vi "EEG.vi"() -> ()   [LabVIEW 2021]
uses:
  <vilib>/Instr/_visa.llb/VISA Configure Serial Port (Instr).vi
panel:
  out "FFT X1 10":cluster{dbl, dbl, dbl[]}(graph)
  out "FFT X7":cluster{dbl, dbl, dbl[]}(graph)
  out "FFT X8":cluster{dbl, dbl, dbl[]}(graph)
  out "FFT X6":cluster{dbl, dbl, dbl[]}(graph)
  out "FFT X5":cluster{dbl, dbl, dbl[]}(graph)
  out "FFT X3":cluster{dbl, dbl, dbl[]}(graph)
  out "Frecuencia Corte Alto":dbl
  in  "Frecuencia Corte Alto":dbl(knob) scale=4.0..45.0
  out "Canal 9":dynamicdata(graph)
  out "Canal 7":dynamicdata(graph)
  out "Canal 8":dynamicdata(graph)
  out "Canal 6":dynamicdata(graph)
  out "Canal 5":dynamicdata(graph) caption="Canal 1"
  out "E9S":dbl[](array[numeric])
  out "E8S":dbl[](array[numeric])
  out "E7S":dbl[](array[numeric])
  out "E6S":dbl[](array[numeric])
  out "E5S":dbl[](array[numeric])
  out "error IO":errorcluster
  out "E4S":dbl[](array[numeric])
  out "E3S":dbl[](array[numeric])
  out "E2S":dbl[](array[numeric])
  out "E1S":dbl[](array[numeric])
  out "DIRECCION 9":string
  out "VALIDADO 2":bool caption="VALIDADO"
  out "FFT X1 4":cluster{dbl, dbl, dbl[]}(graph)
  out "Canal 3":dynamicdata(graph)
  out "Canal 4":dynamicdata(graph)
  out "FFT X4":cluster{dbl, dbl, dbl[]}(graph)
  out "FFT X2":cluster{dbl, dbl, dbl[]}(graph)
  out "Canal 2":dynamicdata(graph)
  out "FFT X1":cluster{dbl, dbl, dbl[]}(graph)
  out "Canal 1":dynamicdata(graph)
  in  "stop":bool
  in  "ADQUIRIR":bool
  out "VALIDADO":bool
  out "DIRECCION 8":string
  out "DIRECCION 7":string
  out "DIRECCION 6":string
  out "DIRECCION 5":string
  out "DIRECCION 4":string
  out "DIRECCION 3":string
  out "DIRECCION 2":string
  out "DIRECCION 1":string
  in  "DETECTAR":bool
  in  "PUERTO COM":refnum<visa-resource-name>
  # "INSTITUTO POLITÉCNICO NACIONAL\nUNIDAD PROFESIONAL INTERDISCIPLINARIA DE INGENIERIA CAMPUS HIDALGO\n\nINTERFAZ EEG"
  # "Direcciones detectadas"
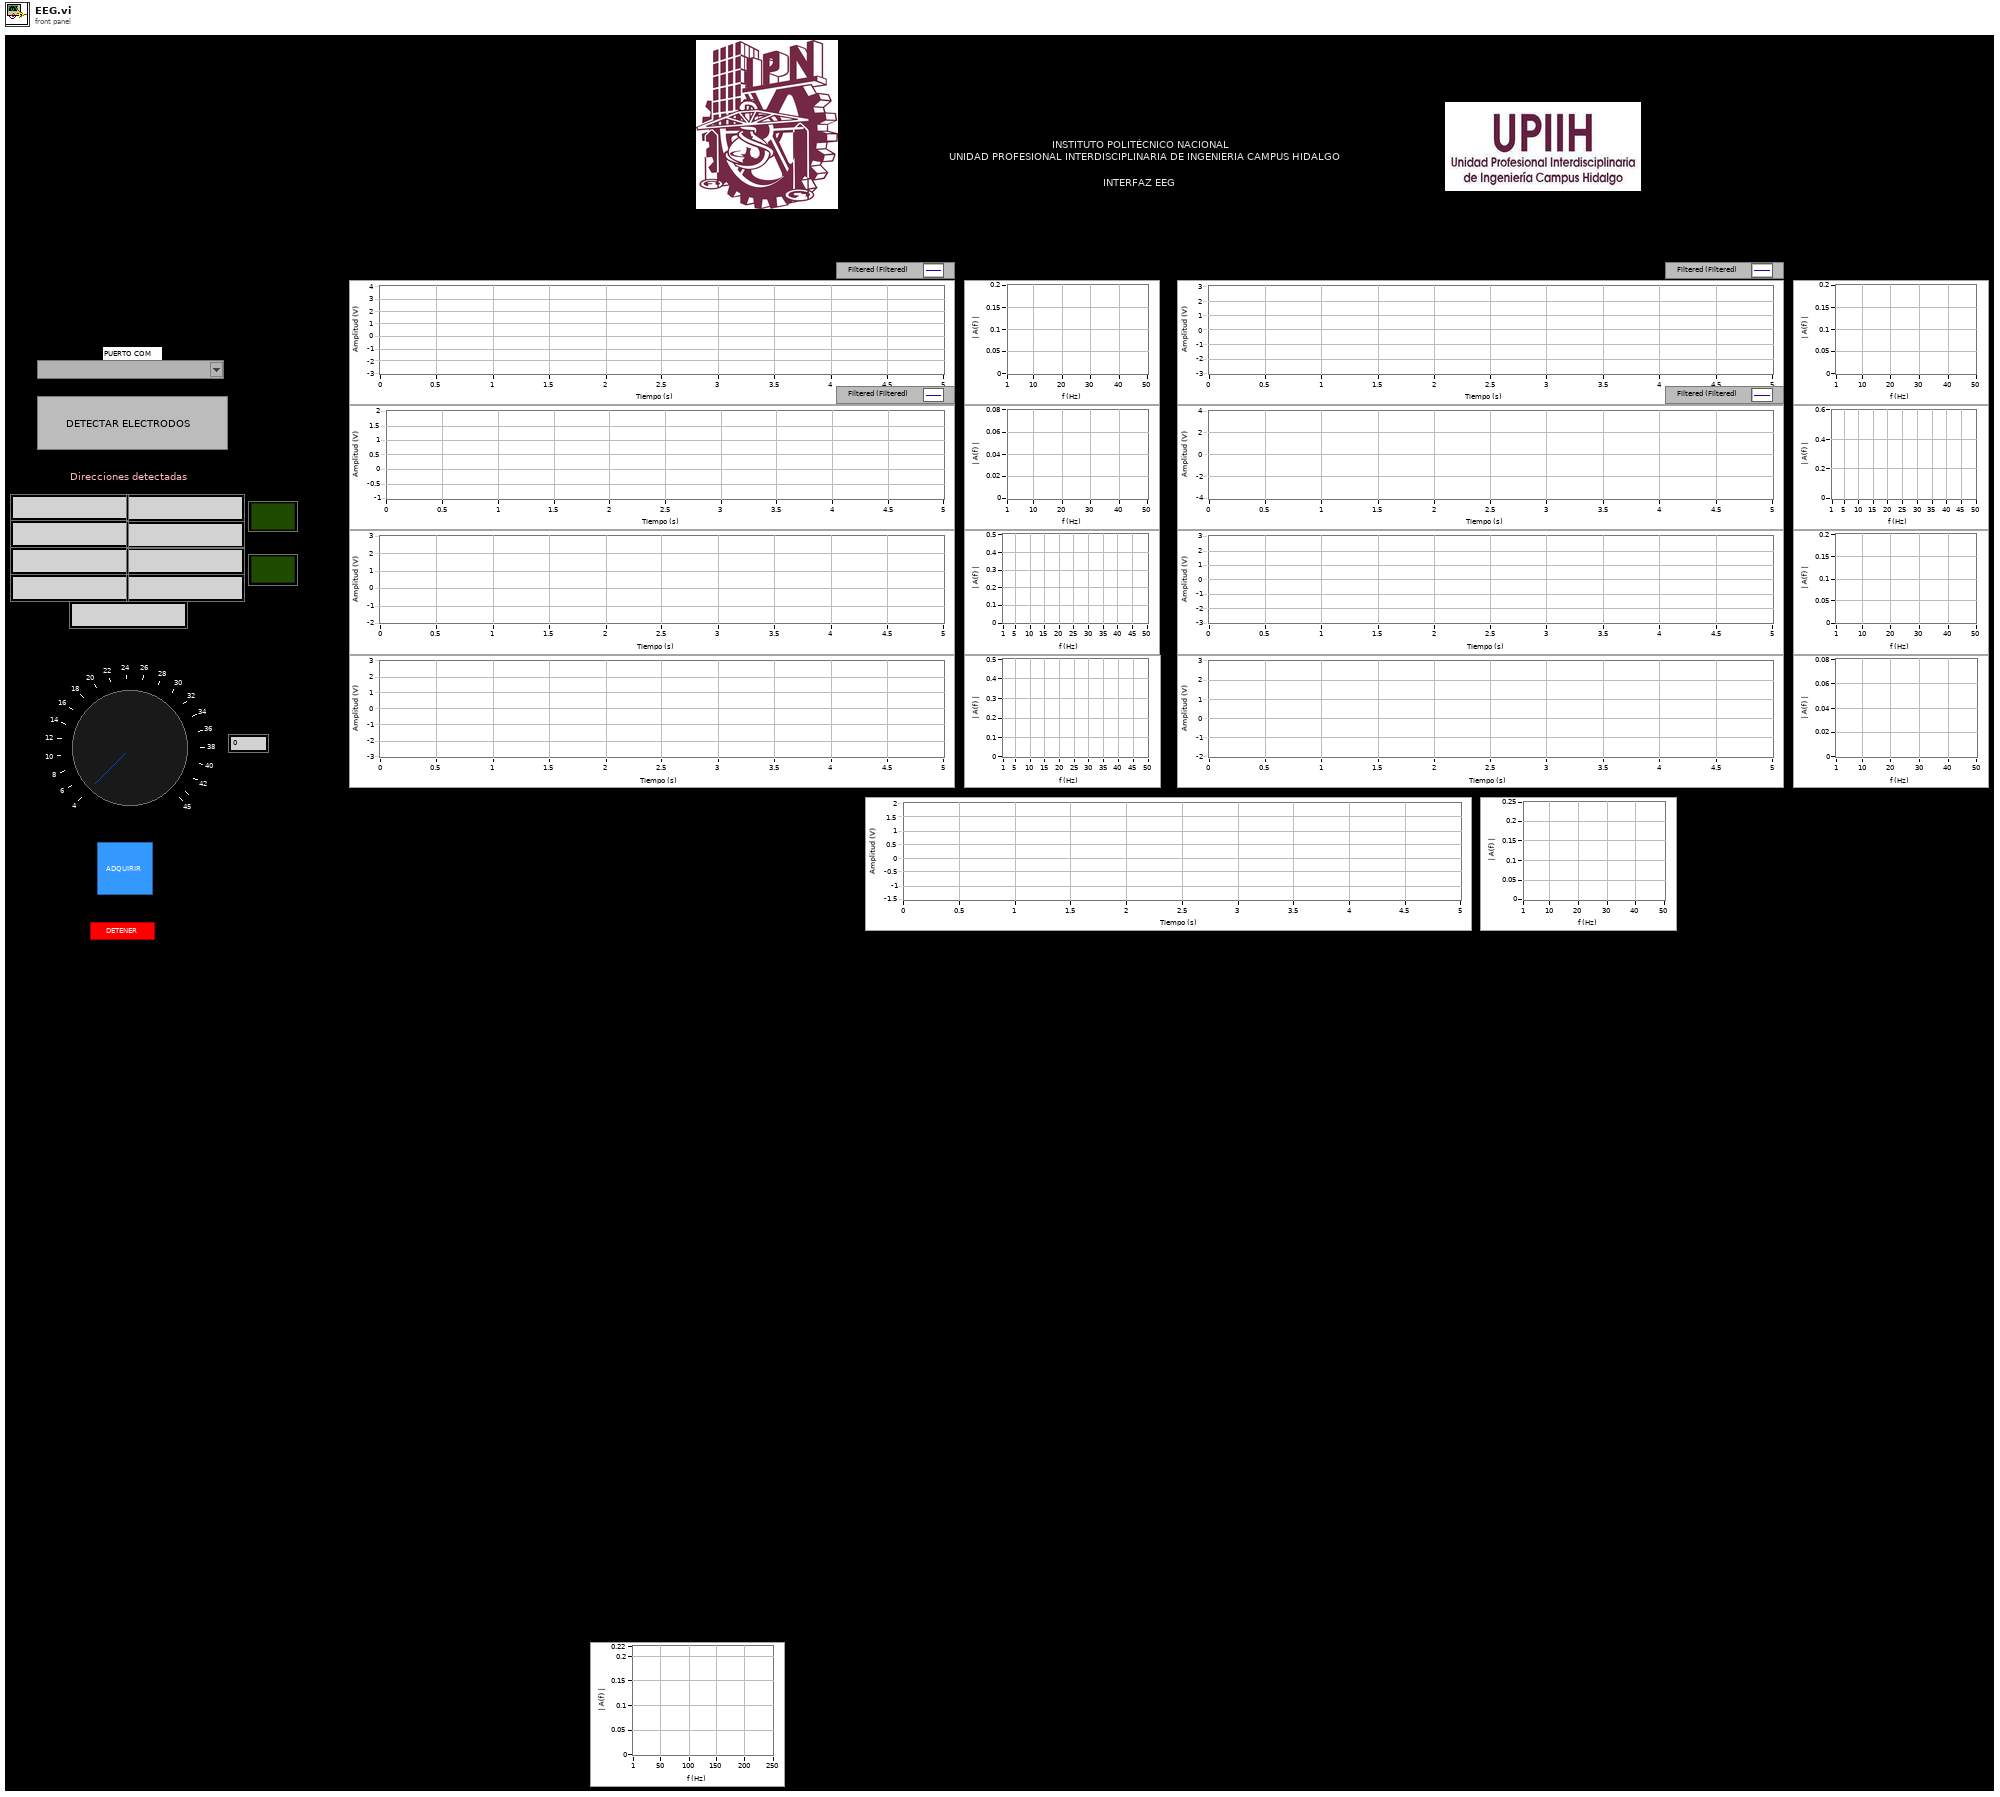
[diagram p1: front panel]
types:
  T1 = cluster{dbl, dbl, dbl, dbl, dbl, dbl, dbl, dbl, dbl}
  T2 = cluster{dbl, dbl, dbl, dbl, dbl, dbl, dbl, dbl, dbl}[]
  T3 = cluster{"Numeric out":dbl, "Numeric 2 out":dbl, "Numeric 3 out":dbl, "Numeric 4 out":dbl, "Numeric 5 out":dbl, "Numeric 6 out":dbl, "Numeric 7 out":dbl, "Numeric 8 out":dbl, "Numeric 9 out":dbl}
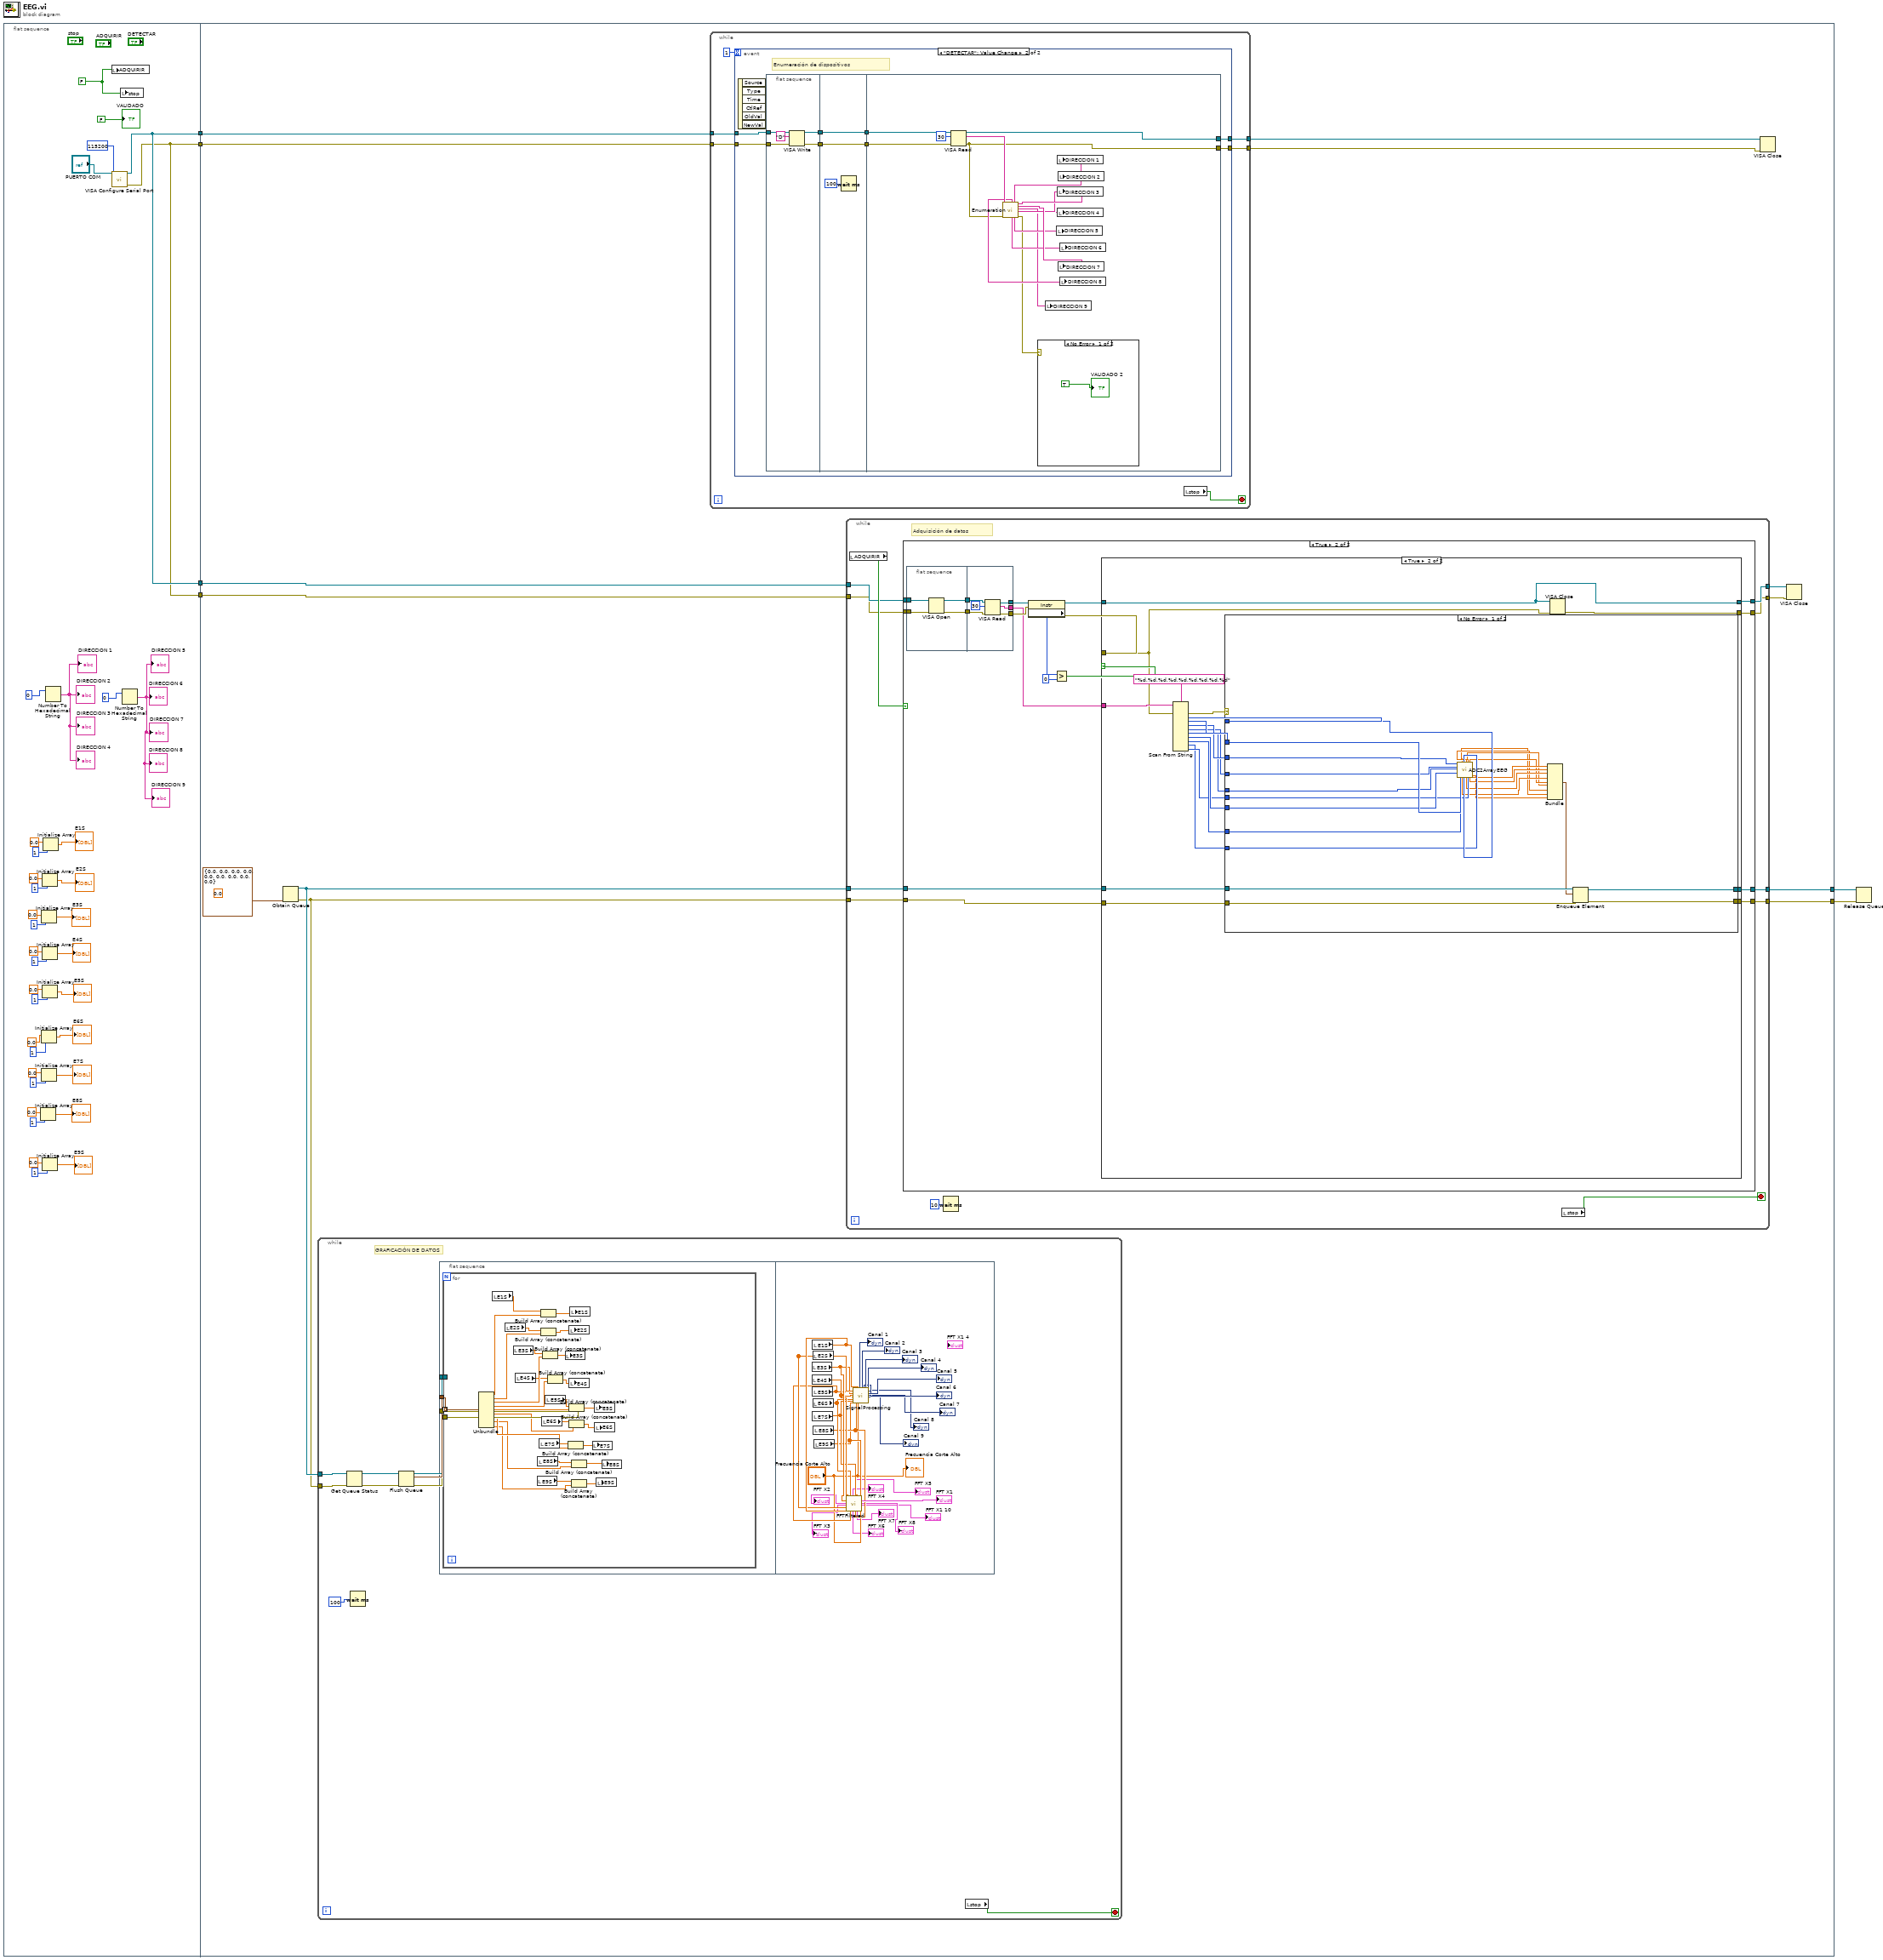
[diagram p0: block diagram]
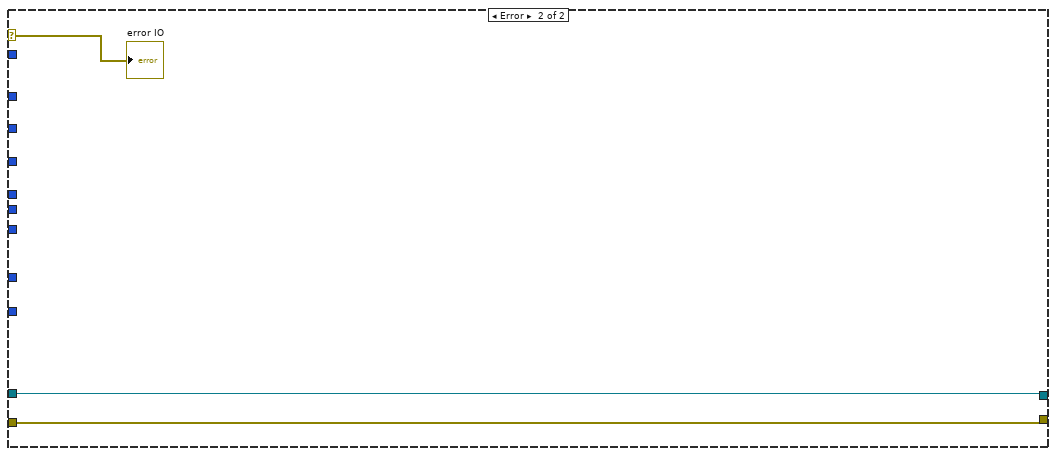
[diagram p4: hidden frame]
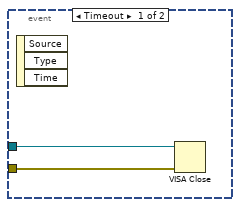
[diagram p5: hidden frame]
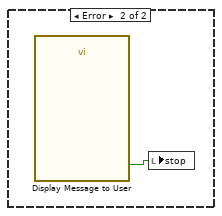
[diagram p6: hidden frame]
diagram:
  n1 = flat-sequence {
    tunnel: [w36] -> w6
    tunnel: [w35] -> w5
    tunnel: [w36] -> w4
    tunnel: [w35] -> w3
    tunnel: w6 -> [w56]
    tunnel: w5 -> [w55]
    tunnel: w4 -> [w52]
    tunnel: w3 -> [w51]
    tunnel: [w48] -> w2
    tunnel: [w47] -> w1
    frame #0 {
      w42 = FALSE
      n2 = Initialize Array(0.0 ("element"), 1 ("dimension size")) -> (→"E8S":dbl[])
      n3 = Initialize Array(0.0 ("element"), 1 ("dimension size")) -> (→"E6S":dbl[])
      n4 = Initialize Array(0.0 ("element"), 1 ("dimension size")) -> (→"E7S":dbl[])
      n5 = Initialize Array(0.0 ("element"), 1 ("dimension size")) -> (→"E3S":dbl[])
      n6 = Initialize Array(0.0 ("element"), 1 ("dimension size")) -> (→"E4S":dbl[])
      n7 = Initialize Array(0.0 ("element"), 1 ("dimension size")) -> (→"E2S":dbl[])
      n8 = Initialize Array(0.0 ("element"), 1 ("dimension size")) -> (→"E5S":dbl[])
      n9 = Initialize Array(0.0 ("element"), 1 ("dimension size")) -> (→"E9S":dbl[])
      n10 = Initialize Array(0.0 ("element"), 1 ("dimension size")) -> (→"E1S":dbl[])
      n11 = Number To Hexadecimal String(2:0) -> (0:→"DIRECCION 3" →"DIRECCION 1" →"DIRECCION 2" →"DIRECCION 4":string)  [unwired: 1 in]
      n12 = local write "ADQUIRIR"(w42) -> ()
      n13 = call-poly "VISA Configure Serial Port"("VISA resource name"="PUERTO COM", "baud rate (9600)"=u32 115200) -> ("VISA resource name out"=w36:refnum<visa-resource-name>, "error out"=w35:errorcluster)  [unwired: 12 in]
      n14 = local write "stop"(w42) -> ()
      n15 = Number To Hexadecimal String(2:0) -> (0:→"DIRECCION 5" →"DIRECCION 6" →"DIRECCION 7" →"DIRECCION 8" →"DIRECCION 9":string)  [unwired: 1 in]
      "VALIDADO" <- FALSE
    }
    frame #1 {
      (unwired) 0.0
      n16 = Obtain Queue(element data type=T1 {0.0, 0.0, 0.0, 0.0, 0.0, 0.0, 0.0, 0.0, 0.0}) -> (queue out=w45:refnum<queue>, error out=w44:errorcluster)  [unwired: 4 in, 1 out]
      n17 = while {
        tunnel: w45 -> [w64]
        tunnel: w44 -> [w63]
        stop <- w65 stop-if-true
        # "GRAFICACIÓN DE DATOS"
        n18 = Get Queue Status(queue=w64, error in (no error)=w63) -> (queue out=w62:refnum<queue>, error out=w61:errorcluster)  [unwired: 1 in, 6 out]
        n19 = Wait (ms)(milliseconds to wait=u32 100) -> ()  [unwired: 1 out]
        n20 = Flush Queue(queue=w62, error in (no error)=w61) -> (queue out=w59:refnum<queue>, remaining elements=w60:T2, error out=w58:errorcluster)
        n21 = flat-sequence {
          tunnel: w60 -> [w66]
          tunnel: w59 -> [w67]
          tunnel: w58 -> [w68]
          frame #0 {
            n22 = for {
              tunnel: w66 -> [w96] mode=indexing
              tunnel: w68 -> [_]
              tunnel: w67 -> [_]
              n23 = Unbundle(w96) -> (w95:dbl, w90:dbl, w89:dbl, w85:dbl, w83:dbl, w78:dbl, w76:dbl, w72:dbl, w70:dbl)
              n24 = local read "E1S"() -> (w94:dbl[])
              n25 = local read "E2S"() -> (w91:dbl[])
              n26 = local read "E3S"() -> (w87:dbl[])
              n27 = local read "E4S"() -> (w86:dbl[])
              n28 = local read "E9S"() -> (w71:dbl[])
              n29 = local read "E8S"() -> (w74:dbl[])
              n30 = local read "E7S"() -> (w77:dbl[])
              n31 = Build Array (concatenate)(w94, w95) -> (w93:dbl[])
              n32 = Build Array (concatenate)(w91, w90) -> (w92:dbl[])
              n33 = local read "E6S"() -> (w80:dbl[])
              n34 = Build Array (concatenate)(w87, w89) -> (w88:dbl[])
              n35 = local read "E5S"() -> (w81:dbl[])
              n36 = Build Array (concatenate)(w86, w85) -> (w84:dbl[])
              n37 = local write "E3S"(w88) -> ()
              n38 = Build Array (concatenate)(w77, w76) -> (w75:dbl[])
              n39 = Build Array (concatenate)(w81, w83) -> (w82:dbl[])
              n40 = local write "E2S"(w92) -> ()
              n41 = local write "E4S"(w84) -> ()
              n42 = Build Array (concatenate)(w80, w78) -> (w79:dbl[])
              n43 = local write "E1S"(w93) -> ()
              n44 = Build Array (concatenate)(w74, w72) -> (w73:dbl[])
              n45 = Build Array (concatenate)(w71, w70) -> (w69:dbl[])
              n46 = local write "E7S"(w75) -> ()
              n47 = local write "E5S"(w82) -> ()
              n48 = local write "E6S"(w79) -> ()
              n49 = local write "E9S"(w69) -> ()
              n50 = local write "E8S"(w73) -> ()
            }
          }
          frame #1 {
            n51 = local read "E3S"() -> (w112:dbl[])
            n52 = local read "E4S"() -> (w111:dbl[])
            n53 = local read "E1S"() -> (w114:dbl[])
            n54 = local read "E5S"() -> (w110:dbl[])
            n55 = local read "E7S"() -> (w108:dbl[])
            n56 = local read "E2S"() -> (w113:dbl[])
            n57 = local read "E6S"() -> (w109:dbl[])
            n58 = local read "E8S"() -> (w107:dbl[])
            n59 = local read "E9S"() -> (w106:dbl[])
            n60 = call "FFTFiltered.vi"("E4S"=w111, "E3S"=w112, "E2S"=w113, "E1S"=w114, "E6S"=w109, "E5S"=w110, "E8S"=w107, "E7S"=w108, "E9S"=w106, "Corte Alto"="Frecuencia Corte Alto") -> ("FFT X2"=→"FFT X2":cluster{dbl, dbl, dbl[]}, "FFT X3"=→"FFT X3":cluster{dbl, dbl, dbl[]}, "FFT X4"=→"FFT X4":cluster{dbl, dbl, dbl[]}, "FFT X6"=→"FFT X6":cluster{dbl, dbl, dbl[]}, "FFT X5"=→"FFT X5":cluster{dbl, dbl, dbl[]}, "FFT X7"=→"FFT X7":cluster{dbl, dbl, dbl[]}, "FFT X1"=→"FFT X1":cluster{dbl, dbl, dbl[]}, "FFT X8"=→"FFT X8":cluster{dbl, dbl, dbl[]}, "FFT X9"=→"FFT X1 10":cluster{dbl, dbl, dbl[]})  [unwired: 1 in]
            n61 = call "SignalProcessing.vi"("E2S"=w113, "E3S"=w112, "E4S"=w111, "E5S"=w110, "E6S"=w109, "E7S"=w108, "E9S"=w106, "E8S"=w107, "E1S"=w114, "Corte Alto"="Frecuencia Corte Alto") -> ("X1"=→"Canal 1":dynamicdata, "X2"=→"Canal 2":dynamicdata, "X6"=→"Canal 6":dynamicdata, "X3"=→"Canal 3":dynamicdata, "X4"=→"Canal 4":dynamicdata, "X8"=→"Canal 8":dynamicdata, "X5"=→"Canal 5":dynamicdata, "X7"=→"Canal 7":dynamicdata, "X9"=→"Canal 9":dynamicdata)  [unwired: 9 in]
            "Frecuencia Corte Alto" <- "Frecuencia Corte Alto"
          }
        }
        n62 = local read "stop"() -> (w65:bool)
      }
      n63 = while {
        tunnel: w56 -> [w220]
        tunnel: w55 -> [w219]
        tunnel: [w217] -> w54
        tunnel: [w216] -> w53
        stop <- w218 stop-if-true
        n64 = event shown="[1] \"DETECTAR\": Value Change" {
          selector: _ -> [_ _]
          dyn-events: _ -> [_ _]
          timeout: 1 -> [_ _]
          tunnel: w220 -> [w223 w231]
          tunnel: w219 -> [w222 w230]
          tunnel: [_ w225] -> w217
          tunnel: [_ w224] -> w216
          event Timeout {
            n65 = event-data() -> ()  [unwired: 1 in, 3 out]
            n66 = VISA Close(VISA resource name=w223, error in (no error)=w222) -> ()  [unwired: 1 out]
          }
          event "DETECTAR": Value Change {
            # "Enumeración de dispositivos"
            n67 = event-data() -> ()  [unwired: 1 in, 6 out]
            n68 = flat-sequence {
              tunnel: w231 -> [w236]
              tunnel: w230 -> [w235]
              tunnel: [w233] -> w229
              tunnel: [w232] -> w228
              tunnel: w229 -> [w238]
              tunnel: w228 -> [w237]
              tunnel: [w238] -> w227
              tunnel: [w237] -> w226
              tunnel: w227 -> [w254]
              tunnel: w226 -> [w255]
              tunnel: [w242] -> w225
              tunnel: [w241] -> w224
              frame #0 {
                n69 = VISA Write(VISA resource name=w236, write buffer="D", error in (no error)=w235) -> (VISA resource name out=w233:refnum<visa-resource-name>, error out=w232:errorcluster)  [unwired: 1 out]
              }
              frame #1 {
                n70 = Wait (ms)(milliseconds to wait=u32 100) -> ()  [unwired: 1 out]
              }
              frame #2 {
                n71 = VISA Read(VISA resource name=w254, byte count=u32 30, error in (no error)=w255) -> (VISA resource name out=w242:refnum<visa-resource-name>, read buffer=w252:string, error out=w241:errorcluster)  [unwired: 1 out]
                n72 = call "Enumeration.vi"("read buffer"=w252, "error in (no error)"=w241) -> ("String 8"=w251:string, "String 6"=w249:string, "String 5"=w248:string, "String"=w244:string, "String 4"=w247:string, "String 7"=w250:string, "String 9"=w240:string, "String 3"=w246:string, "String 2"=w245:string, "error out"=w243:errorcluster)  [unwired: 8 in]
                n73 = case shown="No Error" w243 {
                  frame No Error {
                    "VALIDADO 2" <- TRUE
                  }
                  frame Error {
                    n74 = call "Display Message to User"() -> ("OK"=w257:bool)  [unwired: 10 in, 1 out]
                    n75 = local write "stop"(w257) -> ()
                  }
                }
                n76 = local write "DIRECCION 9"(w240) -> ()
                n77 = local write "DIRECCION 5"(w244) -> ()
                n78 = local write "DIRECCION 1"(w248) -> ()
                n79 = local write "DIRECCION 3"(w246) -> ()
                n80 = local write "DIRECCION 4"(w245) -> ()
                n81 = local write "DIRECCION 2"(w247) -> ()
                n82 = local write "DIRECCION 7"(w250) -> ()
                n83 = local write "DIRECCION 8"(w251) -> ()
                n84 = local write "DIRECCION 6"(w249) -> ()
              }
            }
          }
        }
        n85 = local read "stop"() -> (w218:bool)
      }
      n86 = while {
        tunnel: w52 -> [w134]
        tunnel: w51 -> [w133]
        tunnel: [w132] -> w50
        tunnel: [w131] -> w49
        tunnel: w45 -> [w128]
        tunnel: w44 -> [w127]
        tunnel: [w126] -> w48
        tunnel: [w125] -> w47
        stop <- w130 stop-if-true
        # "Adquisición de datos"
        n87 = local read "ADQUIRIR"() -> (w135:bool)
        n88 = case shown="True" w135 {
          tunnel: w134 -> [w139 w155]
          tunnel: w133 -> [w138 w154]
          tunnel: [w139 w145] -> w132
          tunnel: [w138 w144] -> w131
          tunnel: w128 -> [w137 w143]
          tunnel: w127 -> [w136 w142]
          tunnel: [w137 w141] -> w126
          tunnel: [w136 w140] -> w125
          frame False {
          }
          frame True {
            n89 = flat-sequence {
              tunnel: [w209] -> w157
              tunnel: [w208] -> w156
              tunnel: w155 -> [w207]
              tunnel: w154 -> [w206]
              tunnel: w157 -> [w215]
              tunnel: w156 -> [w214]
              tunnel: [w212] -> w153
              tunnel: [w211] -> w152
              tunnel: [w210] -> w148
              frame #0 {
                n90 = VISA Open(error in (no error)=w206, VISA resource name=w207) -> (VISA resource name=w209:refnum<visa-resource-name>, error out=w208:errorcluster)  [unwired: 3 in]
              }
              frame #1 {
                n91 = VISA Read(VISA resource name=w215, byte count=u32 30, error in (no error)=w214) -> (VISA resource name out=w212:refnum<visa-resource-name>, read buffer=w210:string, error out=w211:errorcluster)  [unwired: 1 out]
              }
            }
            n92 = property class="Instr"(reference=w153, error in=w152) -> (reference out=w146:refnum<visa-resource-name>, error out=w147:errorcluster, "Serial Settings:Number of Bytes at Serial Port"=w151:u32)
            n93 = Greater?(x=w151, y=u32 0) -> (0:w149:bool)
            n94 = case shown="True" w149 {
              tunnel: w148 -> [_ w179]
              tunnel: w147 -> [w160 w168]
              tunnel: [w161 w169] -> w145
              tunnel: w146 -> [w161 w169]
              tunnel: [w160 w168] -> w144
              tunnel: w143 -> [w159 w165]
              tunnel: w142 -> [w158 w164]
              tunnel: [w159 w163] -> w141
              tunnel: [w158 w162] -> w140
              frame False {
              }
              frame True {
                n95 = Scan From String(format string="%d,%d,%d,%d,%d,%d,%d,%d,%d", input string=w179, error in=w168) -> (error out=w177:errorcluster, output 1=w176:i32, output 2=w175:i32, output 3=w174:i32, output 4=w173:i32, output 5=w172:i32, output 6=w171:i32, output 7=w170:i32, output 8=w166:i32, output 9=w167:i32)  [unwired: 10 in, 2 out]
                n96 = case shown="No Error" w177 {
                  selector: w177 -> [_ w205]
                  tunnel: w176 -> [w202 _]
                  tunnel: w175 -> [w201 _]
                  tunnel: w174 -> [w200 _]
                  tunnel: w173 -> [w199 _]
                  tunnel: w172 -> [w198 _]
                  tunnel: w171 -> [w197 _]
                  tunnel: w170 -> [w196 _]
                  tunnel: w166 -> [w195 _]
                  tunnel: w167 -> [w194 _]
                  tunnel: w165 -> [w193 w204]
                  tunnel: w164 -> [w192 w203]
                  tunnel: [w191 w204] -> w163
                  tunnel: [w190 w203] -> w162
                  frame No Error {
                    n97 = call "ADC2ArrayEEG.vi"("Numeric 6"=w200, "Numeric 5"=w199, "Numeric 4"=w198, "Numeric 3"=w197, "Numeric 7"=w201, "Numeric 2"=w196, "Numeric 8"=w202, "Numeric"=w195, "Numeric 9"=w194) -> ("Numeric 8 out"=w182:dbl, "Numeric 4 out"=w186:dbl, "Numeric 7 out"=w183:dbl, "Numeric 3 out"=w187:dbl, "Numeric 6 out"=w184:dbl, "Numeric 5 out"=w185:dbl, "Numeric 2 out"=w188:dbl, "Numeric 9 out"=w181:dbl, "Numeric out"=w189:dbl)  [unwired: 10 in]
                    n98 = Bundle("Numeric out"=w189, "Numeric 2 out"=w188, "Numeric 3 out"=w187, "Numeric 4 out"=w186, "Numeric 5 out"=w185, "Numeric 6 out"=w184, "Numeric 7 out"=w183, "Numeric 8 out"=w182, "Numeric 9 out"=w181) -> (w180:T3)  [unwired: 1 in]
                    n99 = Enqueue Element(queue=w193, element=w180, error in (no error)=w192) -> (queue out=w191:refnum<queue>, error out=w190:errorcluster)  [unwired: 1 in, 1 out]
                  }
                  frame Error {
                    "error IO" <- w205
                  }
                }
                n100 = VISA Close(VISA resource name=w169, error in (no error)=w168) -> ()  [unwired: 1 out]
              }
            }
          }
        }
        n101 = Wait (ms)(milliseconds to wait=u32 10) -> ()  [unwired: 1 out]
        n102 = local read "stop"() -> (w130:bool)
      }
      n103 = VISA Close(VISA resource name=w54, error in (no error)=w53) -> ()  [unwired: 1 out]
      n104 = VISA Close(VISA resource name=w50, error in (no error)=w49) -> ()  [unwired: 1 out]
    }
  }
  n105 = Release Queue(queue=w2, error in (no error)=w1) -> ()  [unwired: 1 in, 3 out]
